vi "Read Fill color.vi"(9 "Slide in":refnum<class "Slide.lvclass">) -> (3 "Slide out":refnum<class "Slide.lvclass">, 4 "Fill color":u32(colorbox))   [LabVIEW 2014, in "Slide.lvclass"]
uses:
  Slide.lvclass
  Slide.lvclass/Slide.ctl
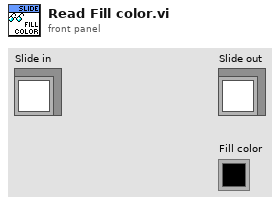
[diagram p1: front panel]
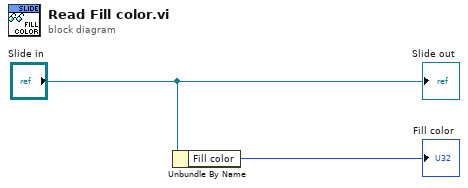
[diagram p0: block diagram]
diagram:
  n1 = Unbundle By Name("Slide in") -> ("Fill color"=→"Fill color":u32)
  "Slide out" <- "Slide in"
